vi "Log.vi"(8 "error in":errorcluster, 9 "Meta Data":string[](array[string]), 10 "String Data":string[](array[string]), 11 "File Splitting Logger in":refnum<class "File Splitting Logger.lvclass">) -> (0 "error out":errorcluster, 3 "File Splitting Logger out":refnum<class "File Splitting Logger.lvclass">)   [LabVIEW 2020, in "File Splitting Logger.lvclass"]
uses:
  File Splitting Logger.lvclass
  File Splitting Logger.lvclass/File Splitting Logger.ctl
  File Logger Interface/File Type Interface.lvclass
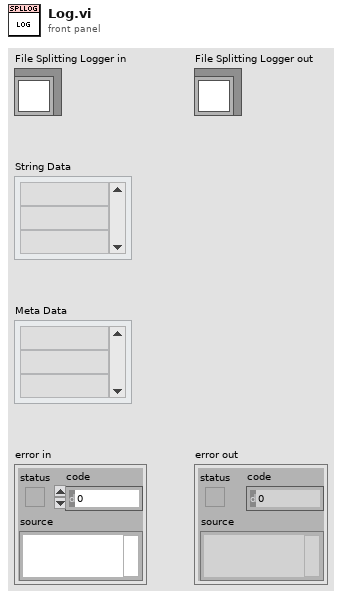
[diagram p1: front panel]
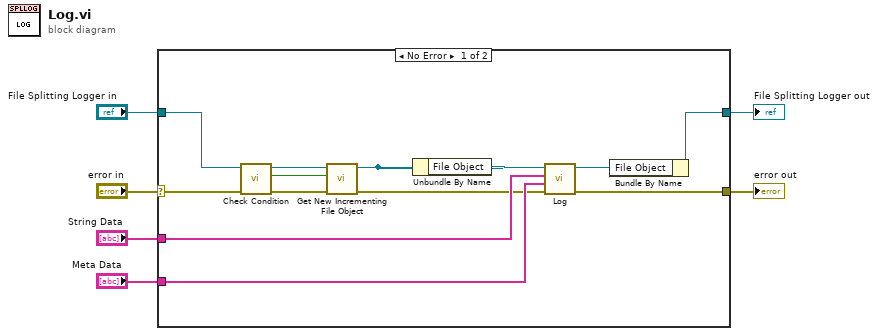
[diagram p0: block diagram]
diagram:
  n1 = case shown="No Error" "error in" {
    selector: "error in" -> [w19 w20]
    tunnel: "File Splitting Logger in" -> [w18 w21]
    tunnel: "String Data" -> [w13 _]
    tunnel: "Meta Data" -> [w12 _]
    tunnel: [w9 w21] -> w2
    tunnel: [w7 w20] -> w1
    frame No Error {
      n2 = call "Check Condition.vi"("error in"=w19, "File Splitting Logger in"=w18) -> ("error out"=w16:errorcluster, "Condition"=w15:bool, "File Splitting Logger out"=w17:refnum<class "File Splitting Logger.lvclass">)  [unwired: 7 in]
      n3 = call "Get New Incrementing File Object.vi"("error in"=w16, "Condition"=w15, "File Splitting Logger in"=w17) -> ("error out"=w8:errorcluster, "File Splitting Logger out"=w10:refnum<class "File Splitting Logger.lvclass">)  [unwired: 7 in]
      n4 = Unbundle By Name(w10) -> ("File Object"=w14:refnum<class "File Type Interface.lvclass">)
      n5 = call-dynamic "Log.vi"("error in"=w8, "Meta Data"=w12, "String Data"=w13, "File Logger Interface in"=w14) -> ("error out"=w7:errorcluster, "File Logger Interface out"=w11:refnum<class "File Type Interface.lvclass">)  [unwired: 6 in]
      n6 = Bundle By Name(cluster=w10, "File Object"=w11) -> (w9:refnum<class "File Splitting Logger.lvclass">)
    }
    frame Error {
    }
  }
  "error out" <- w1
  "File Splitting Logger out" <- w2
